vi "Subtask 4.vi"() -> ()   [LabVIEW 2016, in "LEGO-PMR.lvrbt"]
uses:
  LEGO-PMR.lvrbt
  <vilib>/NXT/Block Support/NXT_InputPort.ctl
  <vilib>/NXT/Block Support/NXT_OutputPort.ctl
  <vilib>/NXT/Dual Mode Library/Sensors/EV3_Ultrasonic_CM.vi
  <vilib>/NXT/NXTIO Xnodes/NXTIONodeSubVIs/NXTStopMotors.vi
  <vilib>/NXT/Dual Mode Library/Display/drawText.vi
  <vilib>/NXT/Dual Mode Library/Sensors/EV3_Color_Reflect.vi
  <vilib>/NXT/Dual Mode Library/Waits/Wait_Num(msec).vi
  <vilib>/NXT/NXTIO Xnodes/NXTIONodeSubVIs/NXTMoveMotors.vi
  <vilib>/NXT/Subs/LVHSConnector.ctl
  <vilib>/NXT/NXTIO Xnodes/AddressXNode/NXTIOAddress.xnode
  <vilib>/NXT/NXTIO Xnodes/NXTIOXNode/NXTIO.xnode
  <vilib>/NXT/LegoClasses/BrickReference/BrickReference.lvclass
panel:
  in  "Metallic Color":string(combo)
  in  "Ceramic Color":string(combo)
  in  "Organic Color":string(combo)
  out "Arm Is Up":bool
  out "Type of Material":string
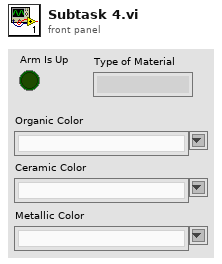
[diagram p1: front panel]
types:
  T1 = typedef "NXT_OutputPort.ctl" = u8
  T2 = typedef "NXT_InputPort.ctl" = u32
  T3 = typedef "LVHSConnector.ctl" = refnum<class "BrickReference.lvclass">
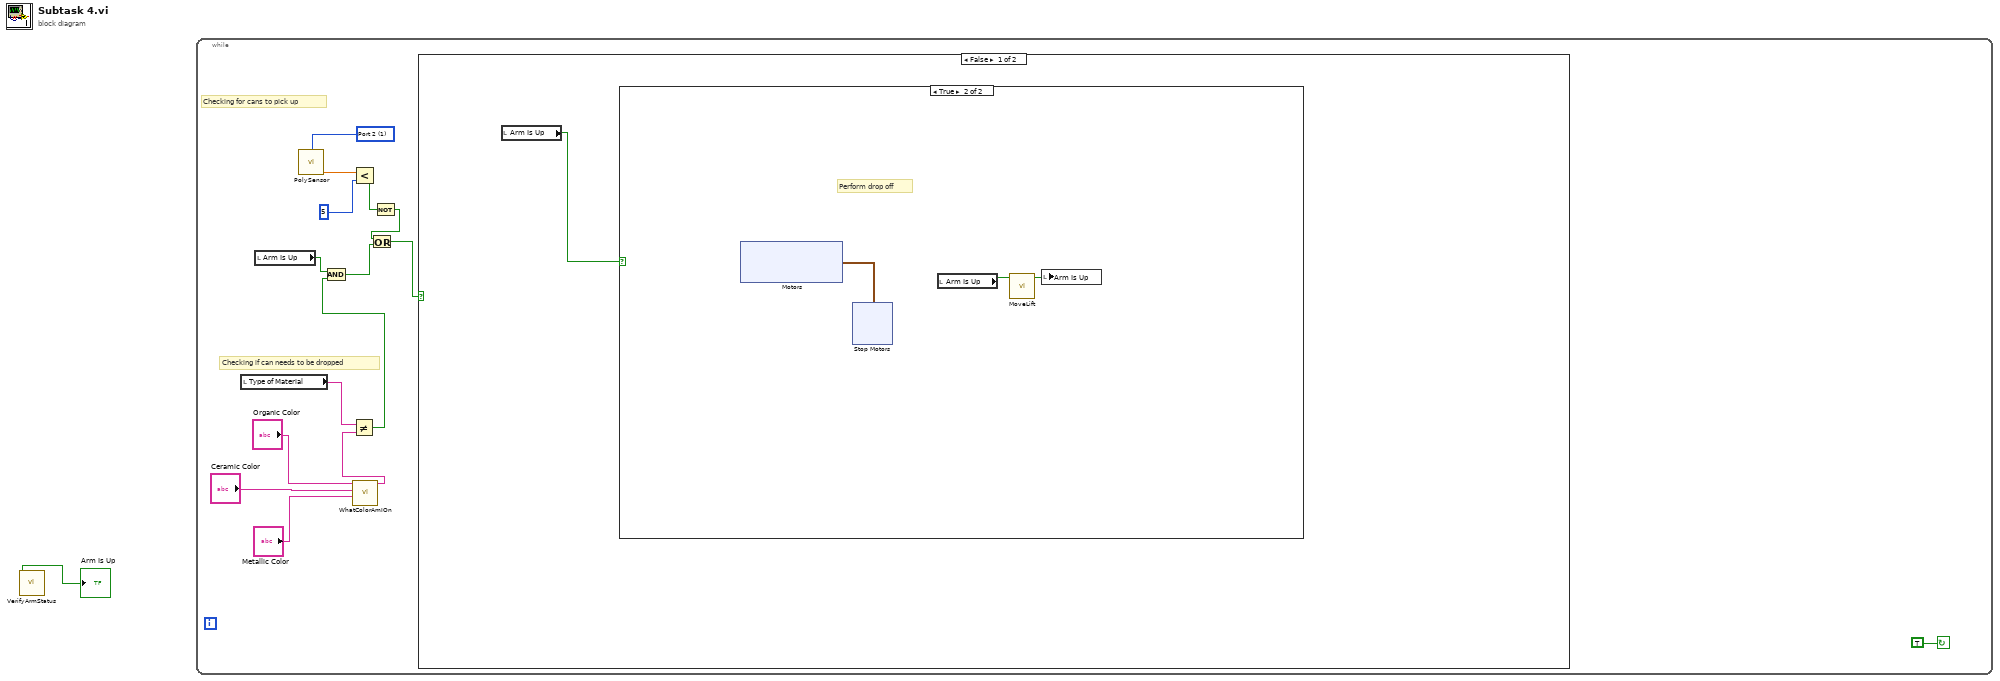
[diagram p0: block diagram]
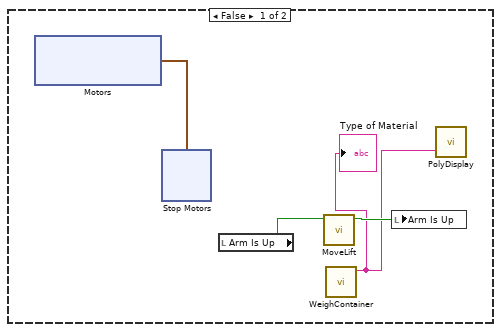
[diagram p2: hidden frame]
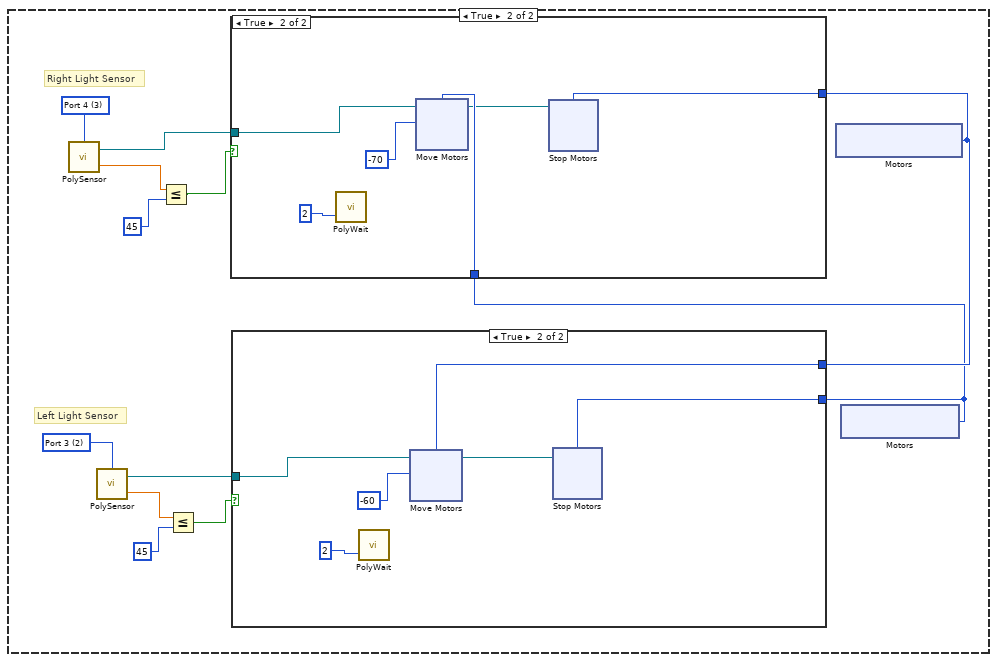
[diagram p3: hidden frame]
diagram:
  n1 = call "VerifyArmStatus.vi"() -> ("Is Arm Up?"=→"Arm Is Up":bool)  [unwired: 11 in]
  n2 = while {
    stop <- TRUE continue-if-true
    w16 = T2 1 items=["Port 1", "Port 2", "Port 3", "Port 4"] ("Port (Port 1)")
    # "Checking for cans to pick up"
    # "Checking if can needs to be dropped"
    n3 = local read "Type of Material"() -> (w8:string)
    n4 = local read "Arm Is Up"() -> (w5:bool)
    n5 = call-poly <vilib>:"PolySensor.vi"("Port (Port 1)"=w16) -> ("Centimeters"=w15:sgl)  [unwired: 2 in, 1 out]
    n6 = Less?(x=w15, y=5) -> (x < y?=w12:bool)
    n7 = call "WhatColorAmIOn.vi"("Metallic Materials Color"="Metallic Color", "Ceramic Materials Color"="Ceramic Color", "Organic Materials Color"="Organic Color") -> ("Drop Off Zone Type"=w7:string)  [unwired: 8 in]
    n8 = Not Equal?(x=w8, y=w7) -> (x != y?=w4:bool)
    n9 = And(x=w5, y=w4) -> (x .and. y?=w3:bool)
    n10 = Not(x=w12) -> (.not. x?=w13:bool)
    n11 = Or(x=w13, y=w3) -> (x .or. y?=w6:bool)
    n12 = case shown="False" w6 {
      frame False {
        n13 = local read "Arm Is Up"() -> (w17:bool)
        n14 = case shown="True" w17 {
          frame False {
            n15 = xnode "Motors"() -> ("Motor"=w21:cluster{"Port":T1, "Port":T1})
            n16 = xnode "Stop Motors"("Motors"=w21) -> ()  [unwired: 1 in, 1 out]
            n17 = local read "Arm Is Up"() -> (w20:bool)
            n18 = call "MoveLift.vi"("Arm is Up?"=w20) -> ("Updated Bool"=w19:bool)  [unwired: 10 in]
            n19 = call "WeighContainer.vi"() -> ("Type"=w18:string)  [unwired: 10 in, 1 out]
            "Type of Material" <- w18
            n20 = local write "Arm Is Up"(w19) -> ()
            n21 = call-poly <vilib>:"PolyDisplay.vi"("Text"=w18) -> ()  [unwired: 3 in, 1 out]
          }
          frame True {
            # "Perform drop off"
            n22 = xnode "Motors"() -> ("Motor"=w30:cluster{"Port":T1, "Port":T1})
            n23 = xnode "Stop Motors"("Motors"=w30) -> ()  [unwired: 1 in, 1 out]
            n24 = local read "Arm Is Up"() -> (w29:bool)
            n25 = call "MoveLift.vi"("Arm is Up?"=w29) -> ("Updated Bool"=w28:bool)  [unwired: 10 in]
            n26 = local write "Arm Is Up"(w28) -> ()
          }
        }
      }
      frame True {
        w47 = T2 3 items=["Port 1", "Port 2", "Port 3", "Port 4"] ("Port (Port 1)")
        w48 = T2 2 items=["Port 1", "Port 2", "Port 3", "Port 4"] ("Port (Port 1)")
        # "Left Light Sensor"
        # "Right Light Sensor"
        n27 = call-poly <vilib>:"PolySensor.vi"("Port (Port 1)"=w47) -> ("Scaled Value"=w41:sgl, "NXT/EV3"=w43:T3)  [unwired: 2 in]
        n28 = call-poly <vilib>:"PolySensor.vi"("Port (Port 1)"=w48) -> ("Scaled Value"=w39:sgl, "NXT/EV3"=w44:T3)  [unwired: 2 in]
        n29 = Less Or Equal?(x=w41, y=45) -> (x <= y?=w42:bool)
        n30 = Less Or Equal?(x=w39, y=45) -> (x <= y?=w37:bool)
        n31 = xnode "Motors"() -> ("Motor"=w46:T1)
        n32 = xnode "Motors"() -> ("Motor"=w45:T1)
        n33 = case shown="True" w42 {
          tunnel: w46 -> [_ w73]
          tunnel: w45 -> [_ w72]
          tunnel: w43 -> [_ w71]
          frame False {
          }
          frame True {
            n34 = call-poly <vilib>:"PolyWait.vi"("Time (100 msec)"=u32 2) -> ()  [unwired: 3 in, 1 out]
            n35 = xnode "Move Motors"("Power/Speed 1"=-70, "Motors"=w72, "NXT/EV3"=w71) -> ("NXT/EV3"=w70:T3)
            n36 = xnode "Stop Motors"("Motors"=w73, "NXT/EV3"=w70) -> ()  [unwired: 1 out]
          }
        }
        n37 = case shown="True" w37 {
          tunnel: w46 -> [_ w55]
          tunnel: w45 -> [_ w54]
          tunnel: w44 -> [_ w53]
          frame False {
          }
          frame True {
            n38 = call-poly <vilib>:"PolyWait.vi"("Time (100 msec)"=u32 2) -> ()  [unwired: 3 in, 1 out]
            n39 = xnode "Move Motors"("Power/Speed 1"=-60, "Motors"=w55, "NXT/EV3"=w53) -> ("NXT/EV3"=w52:T3)
            n40 = xnode "Stop Motors"("Motors"=w54, "NXT/EV3"=w52) -> ()  [unwired: 1 out]
          }
        }
      }
    }
  }
